vi "Get Address Map Element.vi"(2 "niInstr AXI4-Lite address space v1 FPGA in":refnum<class "niInstr AXI4-Lite Address Space v1 FPGA.lvclass">, 5 "index":u8) -> (6 "address map element out":T1)   [LabVIEW 2015, in "niInstr AXI4-Lite Address Space v1 FPGA.lvclass"]
doc: "returns the Address Map Element at the specified <b>index</b>.\n\n<B>Input Parameters</B>\n\n<B>niInstr AXI4-Lite address space v1 FPGA in</B> is the AXI4-Lite address space to use.\n\n<B>index</B> is the index of the Address Map Element to return.\n\n<B>Output Parameters</B>\n\n<B>address map element out</B> is the Address Map Element at the specified index.\n\n<B>address map element out.UID</B> is the unique identifier of the Address Map Element.\n\n<B>address map element out.version</B> is the version of the Address Map Element.\n\n<B>address map element out.oldest compatible version</B> is the oldest version of the address map that is compatible with the current version.\n\n<B>address map element out.instance</B> is the specific instance of the specified address map.\n\n<B>address map element out.number of children</B> is the number of Address Map Elements that are children of the current Address Map Element.\n\n<B>address map element out.offset</B> is the register offset of the Address Map Element on the hardware."
uses:
  <instrlib>/_niInstr/CLIP Adapters/v1/FPGA/AXI4-Lite/Address Space/niInstr AXI4-Lite Address Space v1 FPGA.lvclass
  <instrlib>/_niInstr/Instruction Framework/v1/FPGA/Typedefs/Address Map Element.ctl
  <instrlib>/_niInstr/CLIP Adapters/v1/FPGA/AXI4-Lite/Address Space/niInstr AXI4-Lite Address Space v1 FPGA.lvclass/niInstr AXI4-Lite Address Space v1 FPGA.ctl
  <instrlib>/_niInstr/Instruction Framework/v1/FPGA/Typedefs/niInstr Instruction Framework v1 FPGA.lvlib
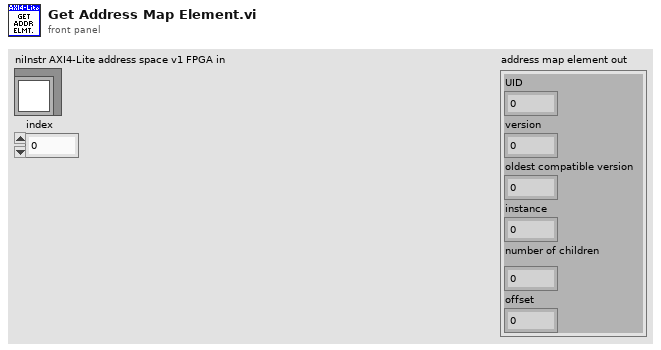
[diagram p1: front panel]
types:
  T1 = typedef "niInstr Instruction Framework v1 FPGA.lvlib/Address Map Element.ctl" = cluster{"UID":u16, "version":u16, "oldest compatible version":u16, "instance":u8, "number of children":u8, "offset":u32}
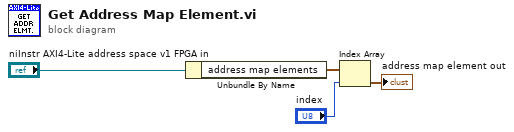
[diagram p0: block diagram]
diagram:
  n1 = Unbundle By Name("niInstr AXI4-Lite address space v1 FPGA in") -> ("address map elements"=w3:T1[])
  n2 = Index Array(array=w3, index="index") -> (element=→"address map element out":T1)
